vi "Lab Panel V5.11.vi"() -> ()   [LabVIEW 2013] (continued)
                n1793 = Not(x=w3340) -> (.not. x?=w3345:bool)
                n1794 = property on="RESULT LAB05-2" class="Bool (strict)"("Visible"=w3343) -> ()  [unwired: 2 in, 2 out]
                n1795 = property on="RESULT LAB05-1" class="Bool (strict)"("Visible"=w3344) -> ()  [unwired: 2 in, 2 out]
                n1796 = Not(x=w3339) -> (.not. x?=w3346:bool)
                n1797 = property on="RESULT LAB04-2" class="Bool (strict)"("Visible"=w3345) -> ()  [unwired: 2 in, 2 out]
                n1798 = Not(x=w3338) -> (.not. x?=w3347:bool)
                n1799 = property on="RESULT LAB04-1" class="Bool (strict)"("Visible"=w3346) -> ()  [unwired: 2 in, 2 out]
                n1800 = property on="RESULT LAB03-2" class="Bool (strict)"("Visible"=w3347) -> ()  [unwired: 2 in, 2 out]
              }
              frame #2 {
                # "disable calibrate if any test running"
                n1801 = Or(x=w3370, y=w3369) -> (x .or. y?=w3363:bool)
                n1802 = Or(x=w3372, y=w3371) -> (x .or. y?=w3365:bool)
                n1803 = Or(x=w3376, y=w3375) -> (x .or. y?=w3367:bool)
                n1804 = Or(x=w3374, y=w3373) -> (x .or. y?=w3366:bool)
                n1805 = Or(x=w3378, y=w3377) -> (x .or. y?=w3368:bool)
                n1806 = Or(x=w3366, y=w3365) -> (x .or. y?=w3364:bool)
                n1807 = Or(x=w3368, y=w3367) -> (x .or. y?=w3362:bool)
                n1808 = Or(x=w3364, y=w3363) -> (x .or. y?=w3361:bool)
                n1809 = Or(x=w3362, y=w3361) -> (x .or. y?=w3360:bool)
                n1810 = case shown="False" w3360 {
                  tunnel: [0 2] -> w3359
                  frame False {
                  }
                  frame True {
                  }
                }
                n1811 = property on="JIG TEST" class="Clust (strict)"("DisabledEnum"=w3359) -> ()  [unwired: 2 in, 2 out]
                n1812 = property on="Network Directory" class="Path"("DisabledEnum"=w3359) -> ()  [unwired: 2 in, 2 out]
                n1813 = property on="MAIL SETTINGS" class="Clust (strict)"("DisabledEnum"=w3359) -> ()  [unwired: 2 in, 2 out]
                n1814 = property on="SET (cal)" class="Bool (strict)"("DisabledEnum"=w3359) -> ()  [unwired: 2 in, 2 out]
                n1815 = property on="ADMIN" class="Bool (strict)"("DisabledEnum"=0) -> ()  [unwired: 2 in, 2 out]
              }
            }
          }
          frame #8 {
            # "drive jigs"
            n1816 = stacked-sequence {
              frame #0 {
                # "jig on"
                n1817 = local read "jig cycle"() -> (w3386:dbl)
                n1818 = property on="JIG TEST" class="Clust (strict)"() -> ("DisabledEnum"=w3383:T16)  [unwired: 2 in, 2 out]
                n1819 = Equal?(x=w3383, y=2) -> (x = y?=w3382:bool)
                n1820 = Equal?(x=w3386, y=0) -> (x = y?=w3384:bool)
                n1821 = And(x=w3384, y=w3382) -> (x .and. y?=w3381:bool)
                n1822 = case shown="True" w3381 {
                  frame False {
                  }
                  frame True {
                    n1823 = local read "run lab01-1"() -> (w3397:bool)
                    n1824 = local read "run lab01-2"() -> (w3396:bool)
                    n1825 = local read "run lab02-1"() -> (w3395:bool)
                    n1826 = local read "run lab02-2"() -> (w3394:bool)
                    n1827 = local read "run lab03-1"() -> (w3393:bool)
                    n1828 = local read "run lab03-2"() -> (w3392:bool)
                    n1829 = local read "run lab04-1"() -> (w3391:bool)
                    n1830 = local read "run lab04-2"() -> (w3390:bool)
                    n1831 = local read "run lab05-1"() -> (w3389:bool)
                    n1832 = local read "run lab05-2"() -> (w3388:bool)
                    n1833 = local write "JIG LAB03-2"(w3392) -> ()
                    n1834 = local write "JIG LAB01-1"(w3397) -> ()
                    n1835 = local write "JIG LAB01-2"(w3396) -> ()
                    n1836 = local write "JIG LAB02-1"(w3395) -> ()
                    n1837 = local write "JIG LAB02-2"(w3394) -> ()
                    n1838 = local write "JIG LAB03-1"(w3393) -> ()
                    n1839 = local write "JIG LAB04-1"(w3391) -> ()
                    n1840 = local write "JIG LAB04-2"(w3390) -> ()
                    n1841 = local write "JIG LAB05-1"(w3389) -> ()
                    n1842 = local write "JIG LAB05-2"(w3388) -> ()
                  }
                }
              }
              frame #1 {
                # "jig off"
                n1843 = local read "jig cycle"() -> (w3404:dbl)
                n1844 = local read "on loops"() -> (w3403:dbl)
                n1845 = property on="JIG TEST" class="Clust (strict)"() -> ("DisabledEnum"=w3402:T16)  [unwired: 2 in, 2 out]
                n1846 = Equal?(x=w3402, y=2) -> (x = y?=w3400:bool)
                n1847 = Equal?(x=w3404, y=w3403) -> (x = y?=w3399:bool)
                n1848 = And(x=w3399, y=w3400) -> (x .and. y?=w3398:bool)
                n1849 = case shown="True" w3398 {
                  frame False {
                  }
                  frame True {
                    w3455 = FALSE
                    w3456 = TRUE
                    w3454 = 2
                    n1850 = local read "SELECT LAB05-2"() -> (w3445:T3)
                    n1851 = local read "SELECT LAB04-2"() -> (w3447:T3)
                    n1852 = local read "SELECT LAB04-1"() -> (w3448:T3)
                    n1853 = local read "SELECT LAB05-1"() -> (w3446:T3)
                    n1854 = local read "SELECT LAB03-2"() -> (w3449:T3)
                    n1855 = local read "SELECT LAB02-1"() -> (w3452:T3)
                    n1856 = local read "SELECT LAB03-1"() -> (w3450:T3)
                    n1857 = local read "SELECT LAB02-2"() -> (w3451:T3)
                    n1858 = local read "SELECT LAB01-2"() -> (w3453:T3)
                    n1859 = local read "run lab05-1"() -> (w3415:bool)
                    n1860 = local read "run lab05-2"() -> (w3414:bool)
                    n1861 = local read "SELECT LAB01-1"() -> (w3457:T3)
                    n1862 = local read "run lab04-2"() -> (w3416:bool)
                    n1863 = local read "run lab04-1"() -> (w3417:bool)
                    n1864 = local read "run lab01-1"() -> (w3433:bool)
                    n1865 = local read "run lab01-2"() -> (w3422:bool)
                    n1866 = local read "run lab03-2"() -> (w3418:bool)
                    n1867 = local read "run lab03-1"() -> (w3419:bool)
                    n1868 = local read "run lab02-1"() -> (w3421:bool)
                    n1869 = local read "run lab02-2"() -> (w3420:bool)
                    n1870 = Equal?(x=w3454, y=w3450) -> (x = y?=w3428:bool)
                    n1871 = Equal?(x=w3454, y=w3449) -> (x = y?=w3427:bool)
                    n1872 = Equal?(x=w3454, y=w3448) -> (x = y?=w3426:bool)
                    n1873 = Equal?(x=w3454, y=w3447) -> (x = y?=w3425:bool)
                    n1874 = Equal?(x=w3454, y=w3446) -> (x = y?=w3424:bool)
                    n1875 = Equal?(x=w3454, y=w3445) -> (x = y?=w3423:bool)
                    n1876 = Equal?(x=w3454, y=w3457) -> (x = y?=w3434:bool)
                    n1877 = Equal?(x=w3454, y=w3452) -> (x = y?=w3430:bool)
                    n1878 = Equal?(x=w3454, y=w3451) -> (x = y?=w3429:bool)
                    n1879 = Equal?(x=w3454, y=w3453) -> (x = y?=w3431:bool)
                    n1880 = And(x=w3425, y=w3416) -> (x .and. y?=w3407:bool)
                    n1881 = And(x=w3428, y=w3419) -> (x .and. y?=w3410:bool)
                    n1882 = And(x=w3426, y=w3417) -> (x .and. y?=w3408:bool)
                    n1883 = And(x=w3423, y=w3414) -> (x .and. y?=w3405:bool)
                    n1884 = And(x=w3429, y=w3420) -> (x .and. y?=w3411:bool)
                    n1885 = And(x=w3427, y=w3418) -> (x .and. y?=w3409:bool)
                    n1886 = And(x=w3424, y=w3415) -> (x .and. y?=w3406:bool)
                    n1887 = And(x=w3431, y=w3422) -> (x .and. y?=w3413:bool)
                    n1888 = And(x=w3434, y=w3433) -> (x .and. y?=w3432:bool)
                    n1889 = And(x=w3430, y=w3421) -> (x .and. y?=w3412:bool)
                    n1890 = Select(t=w3456, s=w3432, f=w3455) -> (s? t:f=w3435:bool)
                    n1891 = Select(t=w3456, s=w3413, f=w3455) -> (s? t:f=w3436:bool)
                    n1892 = Select(t=w3456, s=w3412, f=w3455) -> (s? t:f=w3437:bool)
                    n1893 = Select(t=w3456, s=w3411, f=w3455) -> (s? t:f=w3438:bool)
                    n1894 = Select(t=w3456, s=w3410, f=w3455) -> (s? t:f=w3439:bool)
                    n1895 = Select(t=w3456, s=w3409, f=w3455) -> (s? t:f=w3440:bool)
                    n1896 = Select(t=w3456, s=w3408, f=w3455) -> (s? t:f=w3441:bool)
                    n1897 = Select(t=w3456, s=w3407, f=w3455) -> (s? t:f=w3442:bool)
                    n1898 = Select(t=w3456, s=w3406, f=w3455) -> (s? t:f=w3443:bool)
                    n1899 = Select(t=w3456, s=w3405, f=w3455) -> (s? t:f=w3444:bool)
                    n1900 = local write "JIG LAB03-2"(w3440) -> ()
                    n1901 = local write "JIG LAB02-1"(w3437) -> ()
                    n1902 = local write "JIG LAB02-2"(w3438) -> ()
                    n1903 = local write "JIG LAB01-2"(w3436) -> ()
                    n1904 = local write "JIG LAB03-1"(w3439) -> ()
                    n1905 = local write "JIG LAB01-1"(w3435) -> ()
                    n1906 = local write "JIG LAB05-2"(w3444) -> ()
                    n1907 = local write "JIG LAB04-1"(w3441) -> ()
                    n1908 = local write "JIG LAB05-1"(w3443) -> ()
                    n1909 = local write "JIG LAB04-2"(w3442) -> ()
                  }
                }
              }
            }
          }
          frame #9 {
            # "enable  jig test output if no test busy"
            n1910 = property on="JIG TEST" class="Clust (strict)"() -> ("DisabledEnum"=w3460:T16)  [unwired: 2 in, 2 out]
            n1911 = Equal?(x=w3460, y=0) -> (x = y?=w3458:bool)
            n1912 = case shown="True" w3458 {
              frame False {
              }
              frame True {
                n1913 = local read "JIG TEST"() -> (w3471:T10)
                n1914 = Unbundle(w3471) -> ("LAB01-1"=w3470:bool, "LAB01-2"=w3469:bool, "LAB02-1"=w3468:bool, "LAB02-2"=w3467:bool, "LAB03-1"=w3466:bool, "LAB03-2"=w3465:bool, "LAB04-1"=w3464:bool, "LAB04-2"=w3463:bool, "LAB05-1"=w3462:bool, "LAB05-2"=w3461:bool)
                n1915 = local write "JIG LAB05-1"(w3462) -> ()
                n1916 = local write "JIG LAB05-2"(w3461) -> ()
                n1917 = local write "JIG LAB04-1"(w3464) -> ()
                n1918 = local write "JIG LAB04-2"(w3463) -> ()
                n1919 = local write "JIG LAB03-2"(w3465) -> ()
                n1920 = local write "JIG LAB01-1"(w3470) -> ()
                n1921 = local write "JIG LAB02-1"(w3468) -> ()
                n1922 = local write "JIG LAB03-1"(w3466) -> ()
                n1923 = local write "JIG LAB01-2"(w3469) -> ()
                n1924 = local write "JIG LAB02-2"(w3467) -> ()
              }
            }
          }
          frame #10 {
            # "Drive digital output and reset USB and temperature network if required."
            n1925 = global read "Global display 3.vi" "cycle O/F"() -> (w3481:bool)
            n1926 = local read "O/I  LAB05-2"() -> (w3474:bool)
            n1927 = local read "O/I  LAB05-1"() -> (w3476:bool)
            n1928 = local read "JIG LAB05-2"() -> (w3473:bool)
            n1929 = local read "O/I  LAB04-2"() -> (w3478:bool)
            n1930 = local read "JIG LAB05-1"() -> (w3475:bool)
            n1931 = local read "JIG LAB04-2"() -> (w3477:bool)
            n1932 = local read "O/I  LAB03-1"() -> (w3492:bool)
            n1933 = local read "O/I  LAB04-1"() -> (w3488:bool)
            n1934 = local read "O/I  LAB02-1"() -> (w3496:bool)
            n1935 = local read "O/I  LAB02-2"() -> (w3494:bool)
            n1936 = local read "O/I  LAB03-2"() -> (w3490:bool)
            n1937 = local read "JIG LAB04-1"() -> (w3487:bool)
            n1938 = local read "JIG LAB03-2"() -> (w3489:bool)
            n1939 = local read "O/I  LAB01-2"() -> (w3498:bool)
            n1940 = local read "JIG LAB02-1"() -> (w3495:bool)
            n1941 = local read "JIG LAB02-2"() -> (w3493:bool)
            n1942 = local read "JIG LAB03-1"() -> (w3491:bool)
            n1943 = local read "O/I  LAB01-1"() -> (w3500:bool)
            n1944 = local read "JIG LAB01-2"() -> (w3497:bool)
            n1945 = local read "JIG LAB01-1"() -> (w3499:bool)
            n1946 = case shown="False" w3481 {
              tunnel: [w3581 FALSE] -> w3480
              frame False {
                n1947 = local read "Analog error"() -> (w3580:bool)
                n1948 = local read "Reset Measuring"() -> (w3579:bool)
                n1949 = Or(x=w3579, y=w3580) -> (x .or. y?=w3581:bool)
              }
              frame True {
              }
            }
            n1950 = Build Array(w3493, w3492, w3491, w3490, w3489, w3488, w3487) -> (w3485:bool[])
            n1951 = Build Array(w3500, w3499, w3498, w3497, w3496, w3495, w3494) -> (w3486:bool[])
            n1952 = Build Array(w3478, w3477, w3476, w3475, w3474, w3473, FALSE) -> (w3484:bool[])
            n1953 = Not(x=w3481) -> (.not. x?=w3482:bool)
            n1954 = local read "Simulate"() -> (w3483:bool)
            n1955 = And(x=w3482, y=w3480) -> (x .and. y?=w3479:bool)
            n1956 = stacked-sequence {
              tunnel: w3486 -> [w3504 w3510]
              tunnel: w3485 -> [w3503 w3509]
              tunnel: w3484 -> [w3502 w3508]
              tunnel: w3483 -> [w3501 w3511]
              tunnel: w3479 -> [_ w3512]
              frame #0 {
                # "drive outputs for normal use"
                n1957 = case shown="False" w3501 {
                  tunnel: w3504 -> [w3507 _]
                  tunnel: w3503 -> [w3506 _]
                  tunnel: w3502 -> [w3505 _]
                  frame False {
                    n1958 = call "sub vi - Drive Relays All v6.vi"("Array #2"=w3505, "Array #1"=w3506, "Array #0"=w3507) -> ()  [unwired: 8 in, 1 out]
                  }
                  frame True {
                  }
                }
              }
              frame #1 {
                # "system reset routine"
                n1959 = case shown="True" w3512 {
                  tunnel: w3511 -> [_ w3516]
                  tunnel: w3510 -> [_ w3515]
                  tunnel: w3509 -> [_ w3514]
                  tunnel: w3508 -> [_ w3513]
                  frame False {
                  }
                  frame True {
                    n1960 = stacked-sequence {
                      seq-local: [w3518 _ _] -> [_ w3524 _]
                      tunnel: w3516 -> [_ w3528 _]
                      tunnel: w3515 -> [_ w3527 _]
                      tunnel: w3514 -> [_ w3526 _]
                      tunnel: w3513 -> [_ w3525 _]
                      frame #0 {
                        n1961 = case shown="False" "Auto Reset" {
                          tunnel: [w3521 FALSE] -> w3519
                          frame False {
                            n1962 = Two Button Dialog(message="System reset") -> (T button?=w3521:bool)  [unwired: 2 in]
                          }
                          frame True {
                          }
                        }
                        n1963 = local write "Tab Control 2"(5) -> ()
                        n1964 = Or(x="Auto Reset", y=w3519) -> (x .or. y?=w3518:bool)
                      }
                      frame #1 {
                        n1965 = case shown="True" w3524 {
                          tunnel: w3528 -> [_ w3534]
                          tunnel: w3527 -> [_ w3533]
                          tunnel: w3526 -> [_ w3532]
                          tunnel: w3525 -> [_ w3531]
                          frame False {
                          }
                          frame True {
                            n1966 = stacked-sequence {
                              tunnel: w3534 -> [_ w3552 _]
                              tunnel: bool[] [] -> [w3537 w3551 w3560]
                              tunnel: w3533 -> [_ _ w3559]
                              tunnel: w3532 -> [w3536 _ w3558]
                              tunnel: w3531 -> [w3535 _ w3557]
                              tunnel: 3000 -> [w3538 _ w3556]
                              frame #0 {
                                # "switch off test stations for system reset"
                                n1967 = stacked-sequence {
                                tunnel: w3538 -> [w3542 w3546 w3548]
                                tunnel: w3537 -> [w3541 w3545 w3549]
                                tunnel: w3536 -> [w3540 _ _]
                                tunnel: w3535 -> [w3539 w3544 _]
                                frame #0 {
                                # "drive 1st 7 inputs"
                                n1968 = call "sub vi - Drive Relays All v6.vi"("Array #2"=w3539, "Array #1"=w3540, "Array #0"=w3541) -> ()  [unwired: 8 in, 1 out]
                                n1969 = call "Message Display V1.vi"("Message"="Delay off LAB 01-1 to 02-1", "Delay mS"=w3542) -> ()  [unwired: 10 in]
                                }
                                frame #1 {
                                # "drive 2nd 7 inputs"
                                n1970 = call "sub vi - Drive Relays All v6.vi"("Array #2"=w3544, "Array #1"=w3545, "Array #0"=w3545) -> ()  [unwired: 8 in, 1 out]
                                n1971 = call "Message Display V1.vi"("Message"="Delay off LAB 02-2 to 04-1", "Delay mS"=w3546) -> ()  [unwired: 10 in]
                                }
                                frame #2 {
                                # "drive 3rd 7 inputs"
                                n1972 = call "sub vi - Drive Relays All v6.vi"("Array #2"=w3549, "Array #1"=w3549, "Array #0"=w3549) -> ()  [unwired: 8 in, 1 out]
                                n1973 = call "Message Display V1.vi"("Message"="Delay off LAB 04-2 to 05-2", "Delay mS"=w3548) -> ()  [unwired: 10 in]
                                }
                                }
                              }
                              frame #1 {
                                # "reset all usb modules"
                                n1974 = stacked-sequence {
                                tunnel: w3552 -> [_ w3555]
                                tunnel: w3551 -> [w3554 _]
                                frame #0 {
                                n1975 = call "sub vi - Drive Relays All v6.vi"("Array #2"=bool[] [FALSE, FALSE, FALSE, FALSE, FALSE, FALSE, TRUE], "Array #1"=w3554, "Array #0"=w3554) -> ()  [unwired: 8 in, 1 out]
                                }
                                frame #1 {
                                n1976 = call "Reset Meas v 3.vi"("simulate"=w3555) -> ()  [unwired: 11 in]
                                }
                                }
                              }
                              frame #2 {
                                # "switch test stations back on after reset"
                                n1977 = stacked-sequence {
                                tunnel: w3560 -> [w3564 w3567 _]
                                tunnel: w3559 -> [w3563 w3569 w3574]
                                tunnel: w3556 -> [w3562 w3565 w3571]
                                tunnel: w3558 -> [_ w3568 w3573]
                                tunnel: w3557 -> [_ _ w3570]
                                frame #0 {
                                # "drive 1st 7 inputs"
                                n1978 = call "sub vi - Drive Relays All v6.vi"("Array #2"=w3564, "Array #1"=w3564, "Array #0"=w3563) -> ()  [unwired: 8 in, 1 out]
                                n1979 = call "Message Display V1.vi"("Message"="Delay on LAB 01-1 to 02-1", "Delay mS"=w3562) -> ()  [unwired: 10 in]
                                }
                                frame #1 {
                                # "drive 1st & 2nd outputs"
                                n1980 = call "sub vi - Drive Relays All v6.vi"("Array #2"=w3567, "Array #1"=w3568, "Array #0"=w3569) -> ()  [unwired: 8 in, 1 out]
                                n1981 = call "Message Display V1.vi"("Message"="Delay on LAB 02-2 to 04-1", "Delay mS"=w3565) -> ()  [unwired: 10 in]
                                }
                                frame #2 {
                                n1982 = call "sub vi - Drive Relays All v6.vi"("Array #2"=w3570, "Array #1"=w3573, "Array #0"=w3574) -> ()  [unwired: 8 in, 1 out]
                                n1983 = call "Message Display V1.vi"("Message"="Delay on LAB 04-2 to 05-2", "Delay mS"=w3571) -> ()  [unwired: 10 in]
                                }
                                }
                              }
                            }
                          }
                        }
                      }
                      frame #2 {
                        w3577 = 0
                        w3578 = FALSE
                        # "set all back to zero"
                        n1984 = local read "Resets Done"() -> (w3576:dbl)
                        n1985 = local write "Reset Measuring"(w3578) -> ()
                        n1986 = local write "Analog error"(w3578) -> ()
                        n1987 = local write "Error USB #0"(w3578) -> ()
                        n1988 = local write "Error USB #1"(w3578) -> ()
                        n1989 = local write "Error USB #2"(w3578) -> ()
                        n1990 = local write "Er USB#0"(w3577) -> ()
                        n1991 = local write "Er USB#1"(w3577) -> ()
                        n1992 = local write "Er USB#2"(w3577) -> ()
                        n1993 = Increment(x=w3576) -> (x+1=→"Resets Done":dbl)
                      }
                    }
                  }
                }
              }
            }
          }
          frame #11 {
            # "get all analog values from USB devices"
            n1994 = local read "on loops"() -> (w3589:dbl)
            n1995 = local read "jig cycle"() -> (w3586:dbl)
            n1996 = Add(x=w3589, y=1) -> (x+y=w3587:dbl)
            n1997 = Equal?(x=w3586, y=1) -> (x = y?=w3583:bool)
            n1998 = Equal?(x=w3586, y=w3587) -> (x = y?=w3585:bool)
            n1999 = Or(x=w3583, y=w3585) -> (x .or. y?=w3584:bool)
            n2000 = global write "Global display 3.vi" "cycle O/F"(w3583) -> ()
            n2001 = case shown="True" w3584 {
              tunnel: w3583 -> [_ w3593]
              frame False {
              }
              frame True {
                n2002 = local read "Simulate"() -> (w3596:bool)
                n2003 = case shown="False" w3596 {
                  tunnel: [w3612 0.3 ("Analog loop time")] -> w3603
                  tunnel: [w3611 dynamicdata[] [] ("array GRAPH")] -> w3602
                  tunnel: [w3610 w3617] -> w3601
                  tunnel: [w3609 w3617] -> w3600
                  tunnel: [w3608 w3617] -> w3599
                  tunnel: [w3607 w3617] -> w3598
                  tunnel: [w3606 w3617] -> w3597
                  tunnel: w3593 -> [_ w3621]
                  tunnel: [w3605 "Ambient Volts"] -> w3592
                  tunnel: [w3604 bool[] []] -> w3591
                  frame False {
                    n2004 = call "sub vi - Read Analog All v9.3.vi"() -> ("Analog loop time"=w3612:dbl, "array GRAPH"=w3611:dynamicdata[], "LAB01"=w3610:T26, "LAB02"=w3609:T27, "LAB03"=w3608:T28, "LAB04"=w3607:T29, "deg C"=w3605:dbl, "USB Error"=w3604:bool[], "LAB05"=w3606:T30)  [unwired: 7 in]
                  }
                  frame True {
                    n2005 = local read "ON amps"() -> (w3615:dbl)
                    n2006 = local read "OFF amps"() -> (w3616:dbl)
                    n2007 = local read "VOLTS"() -> (w3619:dbl)
                    n2008 = local read "PF"() -> (w3618:dbl)
                    n2009 = Select(t=w3615, s=w3621, f=w3616) -> (s? t:f=w3620:dbl)
                    n2010 = Bundle("OFF amps"=w3620, "VOLTS"=w3619, "PF"=w3618, "OFF amps"=w3620, "VOLTS"=w3619, "PF"=w3618) -> (w3617:T31)  [unwired: 1 in]
                  }
                }
                n2011 = local read "Simulate"() -> (w3595:bool)
                n2012 = stacked-sequence {
                  seq-local: [w3626 _ _ _ _ _ _ _] -> [_ _ _ _ _ _ _ _]
                  seq-local: [w3625 _ _ _ _ _ _ _] -> [_ _ _ _ _ _ _ _]
                  seq-local: [w3624 _ _ _ _ _ _ _] -> [_ _ _ _ _ _ _ w3821]
                  tunnel: w3603 -> [_ w3679 _ _ _ _ _ _]
                  tunnel: w3602 -> [_ w3676 _ _ _ _ _ _]
                  tunnel: w3601 -> [_ _ w3706 _ _ _ _ _]
                  tunnel: w3600 -> [_ _ _ w3734 _ _ _ _]
                  tunnel: w3599 -> [_ _ _ _ w3762 _ _ _]
                  tunnel: w3598 -> [_ _ _ _ _ w3790 _ _]
                  tunnel: w3597 -> [_ _ _ _ _ _ w3818 _]
                  tunnel: w3595 -> [_ _ w3705 w3733 w3761 w3789 w3817 w3823]
                  tunnel: T14 {"1  (A) cal"=1.0, "1 (V) cal"=1.0, "1 (PF) cal"=1.0, "1 (TL) cal"=1.0, "1 (TN) cal"=1.0, "2 (A) cal"=1.0, "2 (V) cal"=1.0, "2 (PF) cal"=1.0, "2 (TL) cal"=1.0, "2 (TN) cal"=1.0} ("CAL LAB01") -> [_ _ w3704 w3732 w3760 w3788 w3816 _]
                  tunnel: w3592 -> [_ _ _ _ _ _ _ w3822]
                  tunnel: w3591 -> [w3629 _ _ _ _ _ _ _]
                  frame #0 {
                    n2013 = Index Array(array=w3629, index=2) -> (element=w3624:bool)
                    n2014 = Index Array(array=w3629, index=1) -> (element=w3625:bool)
                    n2015 = Index Array(array=w3629, index=0) -> (element=w3626:bool)
                    n2016 = local write "Error USB #2"(w3624) -> ()
                    n2017 = local write "Error USB #0"(w3626) -> ()
                    n2018 = local write "Error USB #1"(w3625) -> ()
                    n2019 = stacked-sequence {
                      tunnel: w3626 -> [w3633 _ _ _]
                      tunnel: w3625 -> [_ w3638 _ _]
                      tunnel: 0 -> [w3632 w3637 w3642 _]
                      tunnel: w3624 -> [_ _ w3643 _]
                      frame #0 {
                        n2020 = case shown="True" w3633 {
                          tunnel: w3632 -> [w3634 _]
                          frame False {
                            n2021 = local write "Er USB#0"(w3634) -> ()
                          }
                          frame True {
                            n2022 = local read "Er USB#0"() -> (w3636:dbl)
                            n2023 = Increment(x=w3636) -> (x+1=→"Er USB#0":dbl)
                          }
                        }
                      }
                      frame #1 {
                        n2024 = case shown="True" w3638 {
                          tunnel: w3637 -> [w3639 _]
                          frame False {
                            n2025 = local write "Er USB#1"(w3639) -> ()
                          }
                          frame True {
                            n2026 = local read "Er USB#1"() -> (w3641:dbl)
                            n2027 = Increment(x=w3641) -> (x+1=→"Er USB#1":dbl)
                          }
                        }
                      }
                      frame #2 {
                        n2028 = case shown="True" w3643 {
                          tunnel: w3642 -> [w3644 _]
                          frame False {
                            n2029 = local write "Er USB#2"(w3644) -> ()
                          }
                          frame True {
                            n2030 = local read "Er USB#2"() -> (w3646:dbl)
                            n2031 = Increment(x=w3646) -> (x+1=→"Er USB#2":dbl)
                          }
                        }
                      }
                      frame #3 {
                        w3652 = 5
                        n2032 = local read "Er USB#2"() -> (w3653:dbl)
                        n2033 = local read "Er USB#0"() -> (w3655:dbl)
                        n2034 = local read "Er USB#1"() -> (w3654:dbl)
                        n2035 = Greater Or Equal?(x=w3655, y=w3652) -> (x >= y?=w3650:bool)
                        n2036 = Greater Or Equal?(x=w3654, y=w3652) -> (x >= y?=w3649:bool)
                        n2037 = Greater Or Equal?(x=w3653, y=w3652) -> (x >= y?=w3648:bool)
                        n2038 = Or(x=w3650, y=w3649) -> (x .or. y?=w3651:bool)
                        n2039 = Or(x=w3651, y=w3648) -> (x .or. y?=→"Analog error":bool)
                      }
                    }
                  }
                  frame #1 {
                    # "display graph data on ADM page"
                    n2040 = local write "AI"(TRUE) -> ()
                    n2041 = global write "Global 1.vi" "RATE(Hz)"("RATE (Hz)") -> ()
                    n2042 = global write "Global 1.vi" "SAMPLES"("SAMPLES") -> ()
                    n2043 = Index Array(array=w3676, index=6) -> (element=→"LAB04-1 (GRAPH)":dynamicdata)
                    n2044 = Index Array(array=w3676, index=7) -> (element=→"LAB04-2 (GRAPH)":dynamicdata)
                    n2045 = Index Array(array=w3676, index=9) -> (element=→"LAB05-2 (GRAPH)":dynamicdata)
                    n2046 = Index Array(array=w3676, index=8) -> (element=→"LAB05-1 (GRAPH)":dynamicdata)
                    n2047 = Index Array(array=w3676, index=5) -> (element=→"LAB03-2 (GRAPH)":dynamicdata)
                    n2048 = Index Array(array=w3676, index=0) -> (element=→"LAB01-1 (GRAPH)":dynamicdata)
                    n2049 = Index Array(array=w3676, index=1) -> (element=→"LAB01-2 (GRAPH)":dynamicdata)
                    n2050 = Index Array(array=w3676, index=2) -> (element=→"LAB02-1 (GRAPH)":dynamicdata)
                    n2051 = Index Array(array=w3676, index=3) -> (element=→"LAB02-2 (GRAPH)":dynamicdata)
                    n2052 = Index Array(array=w3676, index=4) -> (element=→"LAB03-1 (GRAPH)":dynamicdata)
                    "AI loop time" <- w3679
                  }
                  frame #2 {
                    n2053 = case shown="False" w3705 {
                      tunnel: [w3707 w3708] -> w3703
                      tunnel: w3704 -> [_ w3708]
                      frame False {
                        n2054 = local read "CAL LAB01"() -> (w3707:T14)
                      }
                      frame True {
                      }
                    }
                    n2055 = Unbundle By Name(w3706) -> ("OFF amps"=w3702:dbl, "VOLTS"=w3701:dbl, "PF"=w3700:dbl, "OFF amps"=w3699:dbl, "VOLTS"=w3698:dbl, "PF"=w3697:dbl)
                    n2056 = Unbundle By Name(w3703) -> ("1  (A) cal"=w3696:dbl, "1 (V) cal"=w3695:dbl, "1 (PF) cal"=w3694:dbl, "2 (A) cal"=w3693:dbl, "2 (V) cal"=w3692:dbl, "2 (PF) cal"=w3691:dbl)  [unwired: 4 out]
                    n2057 = Multiply(x=w3702, y=w3696) -> (x*y=w3689:dbl)
                    n2058 = Multiply(x=w3701, y=w3695) -> (x*y=w3688:dbl)
                    n2059 = Multiply(x=w3700, y=w3694) -> (x*y=w3687:dbl)
                    n2060 = Multiply(x=w3699, y=w3693) -> (x*y=w3685:dbl)
                    n2061 = Multiply(x=w3698, y=w3692) -> (x*y=w3684:dbl)
                    n2062 = Multiply(x=w3697, y=w3691) -> (x*y=w3683:dbl)
                    n2063 = local read "SIG LAB01-1"() -> (w3690:T2)
                    n2064 = local read "SIG LAB01-2"() -> (w3686:T2)
                    n2065 = Bundle By Name(cluster=w3690, "AMPS"=w3689, "VOLTS"=w3688, "PF"=w3687) -> (w3682:T2)
                    n2066 = Bundle By Name(cluster=w3686, "AMPS"=w3685, "VOLTS"=w3684, "PF"=w3683) -> (w3681:T2)
                    n2067 = global write "Global display 1.vi" "SIG LAB01-2"(w3681) -> ()
                    n2068 = global write "Global display 1.vi" "SIG LAB01-1"(w3682) -> ()
                    n2069 = local write "SIG LAB01-2"(w3681) -> ()
                    n2070 = local write "SIG LAB01-1"(w3682) -> ()
                  }
                  frame #3 {
                    n2071 = Unbundle By Name(w3734) -> ("OFF amps"=w3730:dbl, "VOLTS"=w3729:dbl, "PF"=w3728:dbl, "OFF amps"=w3727:dbl, "VOLTS"=w3726:dbl, "PF"=w3725:dbl)
                    n2072 = case shown="True" w3733 {
                      tunnel: [w3735 w3736] -> w3731
                      tunnel: w3732 -> [_ w3736]
                      frame False {
                        n2073 = local read "CAL LAB02"() -> (w3735:T15)
                      }
                      frame True {
                      }
                    }
                    n2074 = Unbundle By Name(w3731) -> ("1  (A) cal"=w3724:dbl, "1 (V) cal"=w3723:dbl, "1 (PF) cal"=w3722:dbl, "2 (A) cal"=w3721:dbl, "2 (V) cal"=w3720:dbl, "2 (PF) cal"=w3719:dbl)  [unwired: 4 out]
                    n2075 = Multiply(x=w3730, y=w3724) -> (x*y=w3717:dbl)
                    n2076 = Multiply(x=w3729, y=w3723) -> (x*y=w3716:dbl)
                    n2077 = Multiply(x=w3728, y=w3722) -> (x*y=w3715:dbl)
                    n2078 = Multiply(x=w3727, y=w3721) -> (x*y=w3713:dbl)
                    n2079 = Multiply(x=w3726, y=w3720) -> (x*y=w3712:dbl)
                    n2080 = Multiply(x=w3725, y=w3719) -> (x*y=w3711:dbl)
                    n2081 = local read "SIG LAB02-1"() -> (w3718:T2)
                    n2082 = local read "SIG LAB02-2"() -> (w3714:T2)
                    n2083 = Bundle By Name(cluster=w3718, "AMPS"=w3717, "VOLTS"=w3716, "PF"=w3715) -> (w3710:T2)
                    n2084 = Bundle By Name(cluster=w3714, "AMPS"=w3713, "VOLTS"=w3712, "PF"=w3711) -> (w3709:T2)
                    n2085 = global write "Global display 1.vi" "SIG LAB02-1"(w3710) -> ()
                    n2086 = local write "SIG LAB02-2"(w3709) -> ()
                    n2087 = global write "Global display 1.vi" "SIG LAB02-2"(w3709) -> ()
                    n2088 = local write "SIG LAB02-1"(w3710) -> ()
                  }
                  frame #4 {
                    n2089 = Unbundle By Name(w3762) -> ("OFF amps"=w3758:dbl, "VOLTS"=w3757:dbl, "PF"=w3756:dbl, "OFF amps"=w3755:dbl, "VOLTS"=w3754:dbl, "PF"=w3753:dbl)
                    n2090 = case shown="True" w3761 {
                      tunnel: [w3763 w3764] -> w3759
                      tunnel: w3760 -> [_ w3764]
                      frame False {
                        n2091 = local read "CAL LAB03"() -> (w3763:T14)
                      }
                      frame True {
                      }
                    }
                    n2092 = Unbundle By Name(w3759) -> ("1  (A) cal"=w3752:dbl, "1 (V) cal"=w3751:dbl, "1 (PF) cal"=w3750:dbl, "2 (A) cal"=w3749:dbl, "2 (V) cal"=w3748:dbl, "2 (PF) cal"=w3747:dbl)  [unwired: 4 out]
                    n2093 = Multiply(x=w3758, y=w3752) -> (x*y=w3745:dbl)
                    n2094 = Multiply(x=w3757, y=w3751) -> (x*y=w3739:dbl)
                    n2095 = Multiply(x=w3756, y=w3750) -> (x*y=w3744:dbl)
                    n2096 = Multiply(x=w3755, y=w3749) -> (x*y=w3742:dbl)
                    n2097 = Multiply(x=w3754, y=w3748) -> (x*y=w3741:dbl)
                    n2098 = Multiply(x=w3753, y=w3747) -> (x*y=w3740:dbl)
                    n2099 = local read "SIG LAB03-1"() -> (w3746:T2)
                    n2100 = local read "SIG LAB03-2"() -> (w3743:T2)
                    n2101 = Bundle By Name(cluster=w3746, "AMPS"=w3745, "VOLTS"=w3739, "PF"=w3744) -> (w3738:T2)
                    n2102 = Bundle By Name(cluster=w3743, "AMPS"=w3742, "VOLTS"=w3741, "PF"=w3740) -> (w3737:T2)
                    n2103 = global write "Global display 1.vi" "SIG LAB03-1"(w3738) -> ()
                    n2104 = global write "Global display 1.vi" "SIG LAB03-2"(w3737) -> ()
                    n2105 = local write "SIG LAB03-2"(w3737) -> ()
                    n2106 = local write "SIG LAB03-1"(w3738) -> ()
                  }
                  frame #5 {
                    n2107 = case shown="False" w3789 {
                      tunnel: [w3791 w3792] -> w3787
                      tunnel: w3788 -> [_ w3792]
                      frame False {
                        n2108 = local read "CAL LAB04"() -> (w3791:T14)
                      }
                      frame True {
                      }
                    }
                    n2109 = Unbundle By Name(w3790) -> ("OFF amps"=w3786:dbl, "VOLTS"=w3785:dbl, "PF"=w3784:dbl, "OFF amps"=w3783:dbl, "VOLTS"=w3782:dbl, "PF"=w3781:dbl)
                    n2110 = Unbundle By Name(w3787) -> ("1  (A) cal"=w3780:dbl, "1 (V) cal"=w3779:dbl, "1 (PF) cal"=w3778:dbl, "2 (A) cal"=w3777:dbl, "2 (V) cal"=w3776:dbl, "2 (PF) cal"=w3775:dbl)  [unwired: 4 out]
                    n2111 = Multiply(x=w3786, y=w3780) -> (x*y=w3773:dbl)
                    n2112 = Multiply(x=w3785, y=w3779) -> (x*y=w3772:dbl)
                    n2113 = Multiply(x=w3784, y=w3778) -> (x*y=w3771:dbl)
                    n2114 = Multiply(x=w3783, y=w3777) -> (x*y=w3769:dbl)
                    n2115 = Multiply(x=w3782, y=w3776) -> (x*y=w3768:dbl)
                    n2116 = Multiply(x=w3781, y=w3775) -> (x*y=w3767:dbl)
                    n2117 = local read "SIG LAB04-1"() -> (w3774:T2)
                    n2118 = local read "SIG LAB04-2"() -> (w3770:T2)
                    n2119 = Bundle By Name(cluster=w3774, "AMPS"=w3773, "VOLTS"=w3772, "PF"=w3771) -> (w3766:T2)
                    n2120 = Bundle By Name(cluster=w3770, "AMPS"=w3769, "VOLTS"=w3768, "PF"=w3767) -> (w3765:T2)
                    n2121 = global write "Global display 1.vi" "SIG LAB04-2"(w3765) -> ()
                    n2122 = global write "Global display 1.vi" "SIG LAB04-1"(w3766) -> ()
                    n2123 = local write "SIG LAB04-2"(w3765) -> ()
                    n2124 = local write "SIG LAB04-1"(w3766) -> ()
                  }
                  frame #6 {
                    n2125 = Unbundle By Name(w3818) -> ("OFF amps"=w3814:dbl, "VOLTS"=w3795:dbl, "PF"=w3813:dbl, "OFF amps"=w3812:dbl, "VOLTS"=w3811:dbl, "PF"=w3810:dbl)
                    n2126 = case shown="False" w3817 {
                      tunnel: [w3819 w3820] -> w3815
                      tunnel: w3816 -> [_ w3820]
                      frame False {
                        n2127 = local read "CAL LAB05"() -> (w3819:T14)
                      }
                      frame True {
                      }
                    }
                    n2128 = Unbundle By Name(w3815) -> ("1  (A) cal"=w3809:dbl, "1 (V) cal"=w3808:dbl, "1 (PF) cal"=w3807:dbl, "2 (A) cal"=w3806:dbl, "2 (V) cal"=w3805:dbl, "2 (PF) cal"=w3804:dbl)  [unwired: 4 out]
                    n2129 = Multiply(x=w3814, y=w3809) -> (x*y=w3802:dbl)
                    n2130 = Multiply(x=w3795, y=w3808) -> (x*y=w3801:dbl)
                    n2131 = Multiply(x=w3813, y=w3807) -> (x*y=w3800:dbl)
                    n2132 = Multiply(x=w3812, y=w3806) -> (x*y=w3798:dbl)
                    n2133 = Multiply(x=w3811, y=w3805) -> (x*y=w3797:dbl)
                    n2134 = Multiply(x=w3810, y=w3804) -> (x*y=w3796:dbl)
                    n2135 = local read "SIG LAB05-1"() -> (w3803:T2)
                    n2136 = local read "SIG LAB05-2"() -> (w3799:T2)
                    n2137 = Bundle By Name(cluster=w3803, "AMPS"=w3802, "VOLTS"=w3801, "PF"=w3800) -> (w3794:T2)
                    n2138 = Bundle By Name(cluster=w3799, "AMPS"=w3798, "VOLTS"=w3797, "PF"=w3796) -> (w3793:T2)
                    n2139 = global write "Global display 1.vi" "SIG LAB05-1"(w3794) -> ()
                    n2140 = global write "Global display 1.vi" "SIG LAB05-2"(w3793) -> ()
                    n2141 = local write "SIG LAB05-2"(w3793) -> ()
                    n2142 = local write "SIG LAB05-1"(w3794) -> ()
                  }
                  frame #7 {
                    n2143 = case shown="False" w3821 {
                      tunnel: w3823 -> [w3825 _]
                      tunnel: w3822 -> [w3824 _]
                      frame False {
                        # "update ambient referance temperature"
                        n2144 = case shown="True" w3825 {
                          tunnel: [w3828 100.0] -> w3827
                          frame False {
                            n2145 = local read "TEMP REF cal"() -> (w3828:dbl)
                          }
                          frame True {
                          }
                        }
                        n2146 = local read "Panel #"() -> (w3826:dbl)
                        n2147 = case shown="1" w3826 {
                          tunnel: w3827 -> [_ w3834]
                          tunnel: w3824 -> [_ w3833]
                          frame 0, Default {
                          }
                          frame 1 {
                            n2148 = Multiply(x=w3834, y=w3833) -> (x*y=w3832:dbl)
                            n2149 = Subtract(x=w3832, y=272) -> (x-y=w3830:dbl)
                            "Amb Tp" <- w3830
                            n2150 = local write "Ref deg C"(w3830) -> ()
                          }
                        }
                        "deg C (volts)" <- w3824
                      }
                      frame True {
                      }
                    }
                  }
                }
              }
            }
          }
          frame #12 {
            # "save test data to file"
            n2151 = Get Date/Time In Seconds() -> (seconds since 1Jan1904=w3835:timestamp)
            "File Time Stamp" <- w3835
            n2152 = local read "on loops"() -> (w3854:dbl)
            n2153 = local read "jig cycle"() -> (w3851:dbl)
            n2154 = Format Date/Time String(time format string (%c)="%H:%M%:%S", seconds (now)=w3835) -> (date/time string=w3839:string)  [unwired: 1 in]
            n2155 = Add(x=w3854, y=2) -> (x+y=w3852:dbl)
            n2156 = Build Array(w3839) -> (w3838:string[])
            n2157 = Equal?(x=w3851, y=1) -> (x = y?=w3837:bool)
            n2158 = Equal?(x=w3851, y=w3852) -> (x = y?=w3836:bool)
            n2159 = stacked-sequence {
              tunnel: w3850 -> [w3860 _ _ _ _ _ _ _ _ _]
              tunnel: w3849 -> [_ w3936 _ _ _ _ _ _ _ _]
              tunnel: w3848 -> [_ _ w4016 _ _ _ _ _ _ _]
              tunnel: w3847 -> [_ _ _ w4096 _ _ _ _ _ _]
              tunnel: w3846 -> [_ _ _ _ w4176 _ _ _ _ _]
              tunnel: w3845 -> [_ _ _ _ _ w4256 _ _ _ _]
              tunnel: w3844 -> [_ _ _ _ _ _ w4336 _ _ _]
              tunnel: w3843 -> [_ _ _ _ _ _ _ w4416 _ _]
              tunnel: w3842 -> [_ _ _ _ _ _ _ _ w4496 _]
              tunnel: w3841 -> [_ _ _ _ _ _ _ _ _ w4576]
              tunnel: w3838 -> [w3859 w3940 w4020 w4100 w4180 w4260 w4340 w4420 w4500 w4580]
              tunnel: w3837 -> [w3858 w3939 w4019 w4099 w4179 w4259 w4339 w4419 w4499 w4579]
              tunnel: w3836 -> [w3857 w3938 w4018 w4098 w4178 w4258 w4338 w4418 w4498 w4578]
              tunnel: w3835 -> [w3856 w3937 w4017 w4097 w4177 w4257 w4337 w4417 w4497 w4577]
              frame #0 {
                n2160 = case shown="True" w3860 {
                  tunnel: w3859 -> [_ w3865]
                  tunnel: w3858 -> [_ w3864]
                  tunnel: w3857 -> [_ w3862]
                  tunnel: w3856 -> [_ w3861]
                  frame False {
                  }
                  frame True {
                    n2161 = local read "DISP LAB01-1"() -> (w3866:T4)
                    n2162 = local read "SIG LAB01-1"() -> (w3867:T2)
                    n2163 = local read "ON L01-1"() -> (w3863:cluster{"amps":dbl, "volts":dbl, "pf":dbl})
                    n2164 = Unbundle(w3867) -> ("AMPS"=w3873:dbl, "VOLTS"=w3871:dbl, "PF"=w3870:dbl, "Tmp Live"=w3869:dbl, "Tmp Neut"=w3872:dbl)
                    n2165 = Unbundle(w3866) -> ("CYCLE"=w3868:dbl)  [unwired: 2 out]
                    n2166 = stacked-sequence {
                      tunnel: w3873 -> [w3877 w3896]
                      tunnel: w3872 -> [_ w3895]
                      tunnel: w3871 -> [w3876 w3894]
                      tunnel: w3870 -> [w3875 w3893]
                      tunnel: w3869 -> [_ w3892]
                      tunnel: w3868 -> [_ w3891]
                      tunnel: w3865 -> [_ w3890]
                      tunnel: w3864 -> [w3878 _]
                      tunnel: w3863 -> [w3874 w3888]
                      tunnel: w3862 -> [_ w3889]
                      tunnel: w3861 -> [_ w3884]
                      frame #0 {
                        n2167 = case shown="True" w3878 {
                          tunnel: w3877 -> [_ w3883]
                          tunnel: w3876 -> [_ w3882]
                          tunnel: w3875 -> [_ w3881]
                          tunnel: w3874 -> [_ w3879]
                          frame False {
                          }
                          frame True {
                            n2168 = Bundle(cluster=w3879, "amps"=w3883, "volts"=w3882, "pf"=w3881) -> (w3880:cluster{"amps":dbl, "volts":dbl, "pf":dbl})
                            n2169 = local write "ON L01-1"(w3880) -> ()
                          }
                        }
                      }
                      frame #1 {
                        n2170 = Unbundle(w3888) -> ("amps"=w3887:dbl, "volts"=w3886:dbl, "pf"=w3885:dbl)
                        n2171 = case shown="True" w3889 {
                          tunnel: w3896 -> [_ w3897]
                          tunnel: w3895 -> [_ w3935]
                          tunnel: w3894 -> [_ _]
                          tunnel: w3893 -> [_ _]
                          tunnel: w3892 -> [_ w3934]
                          tunnel: w3891 -> [_ w3933]
                          tunnel: w3890 -> [_ w3901]
                          tunnel: w3887 -> [_ w3898]
                          tunnel: w3886 -> [_ w3930]
                          tunnel: w3885 -> [_ w3929]
                          tunnel: w3884 -> [_ w3899]
                          frame False {
                          }
                          frame True {
                            n2172 = local read "TDMS LAB01-1"() -> (w3932:refnum<k34>)
                            n2173 = Build Array(w3930) -> (w3926:dbl[])
                            n2174 = Build Array(w3929) -> (w3925:dbl[])
                            n2175 = Build Array(w3934) -> (w3924:dbl[])
                            n2176 = Build Array(w3935) -> (w3923:dbl[])
                            n2177 = Build Array(w3898) -> (w3928:dbl[])
                            n2178 = Build Array(w3897) -> (w3927:dbl[])
                            n2179 = Build Array(w3933) -> (w3922:dbl[])
                            n2180 = Build Array("AMPS ON", "AMPS OFF", "VOLTS", "PF", "TEMP Live", "TEMP Neut", "CYCLE") -> (w3906:string[])
                            n2181 = Bundle By Name("Y"=w3928, "t0"=w3899) -> (w3921:waveform(dbl))  [unwired: 1 in]
                            n2182 = Bundle By Name("Y"=w3927, "t0"=w3899) -> (w3920:waveform(dbl))  [unwired: 1 in]
                            n2183 = Bundle By Name("Y"=w3926, "t0"=w3899) -> (w3919:waveform(dbl))  [unwired: 1 in]
                            n2184 = Bundle By Name("Y"=w3925, "t0"=w3899) -> (w3918:waveform(dbl))  [unwired: 1 in]
                            n2185 = Bundle By Name("Y"=w3924, "t0"=w3899) -> (w3917:waveform(dbl))  [unwired: 1 in]
                            n2186 = Bundle By Name("Y"=w3923, "t0"=w3899) -> (w3916:waveform(dbl))  [unwired: 1 in]
                            n2187 = Bundle By Name("Y"=w3922, "t0"=w3899) -> (w3915:waveform(dbl))  [unwired: 1 in]
                            n2188 = Build Array(w3921, w3920, w3919, w3918, w3917, w3916, w3915) -> (w3914:waveform(dbl)[])
                            n2189 = TDMS Write(0:w3932, 5:"TEST VALUES", 7:w3906, 9:w3914) -> (4:w3905:refnum<k34>, 6:w3904:string, 15:w3903:errorcluster)  [unwired: 2 in, 1 out]
                            n2190 = TDMS Write(0:w3905, 5:w3904, 7:"TIME", 9:w3901, 11:w3903) -> (15:w3900:errorcluster)  [unwired: 1 in, 3 out]
                            n2191 = local write "data file error"(w3900) -> ()
                          }
                        }
                      }
                    }
                  }
                }
              }
              frame #1 {
                n2192 = case shown="True" w3936 {
                  tunnel: w3940 -> [_ w3945]
                  tunnel: w3939 -> [_ w3944]
                  tunnel: w3938 -> [_ w3942]
                  tunnel: w3937 -> [_ w3941]
                  frame False {
                  }
                  frame True {
                    n2193 = local read "DISP LAB01-2"() -> (w3946:T4)
                    n2194 = local read "SIG LAB01-2"() -> (w3947:T2)
                    n2195 = local read "ON L01-2"() -> (w3943:cluster{"amps":dbl, "volts":dbl, "pf":dbl})
                    n2196 = Unbundle(w3947) -> ("AMPS"=w3953:dbl, "VOLTS"=w3951:dbl, "PF"=w3950:dbl, "Tmp Live"=w3949:dbl, "Tmp Neut"=w3952:dbl)
                    n2197 = Unbundle(w3946) -> ("CYCLE"=w3948:dbl)  [unwired: 2 out]
                    n2198 = stacked-sequence {
                      tunnel: w3953 -> [w3957 w3976]
                      tunnel: w3952 -> [_ w3975]
                      tunnel: w3951 -> [w3956 w3974]
                      tunnel: w3950 -> [w3955 w3973]
                      tunnel: w3949 -> [_ w3972]
                      tunnel: w3948 -> [_ w3971]
                      tunnel: w3945 -> [_ w3970]
                      tunnel: w3944 -> [w3958 _]
                      tunnel: w3943 -> [w3954 w3968]
                      tunnel: w3942 -> [_ w3969]
                      tunnel: w3941 -> [_ w3964]
                      frame #0 {
                        n2199 = case shown="True" w3958 {
                          tunnel: w3957 -> [_ w3963]
                          tunnel: w3956 -> [_ w3962]
                          tunnel: w3955 -> [_ w3961]
                          tunnel: w3954 -> [_ w3959]
                          frame False {
                          }
                          frame True {
